vi "BuscaTeensy.vi"() -> (4 "VISA resource name out":refnum<visa-resource-name>)   [LabVIEW 2023]
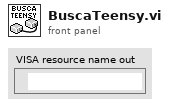
[diagram p1: front panel]
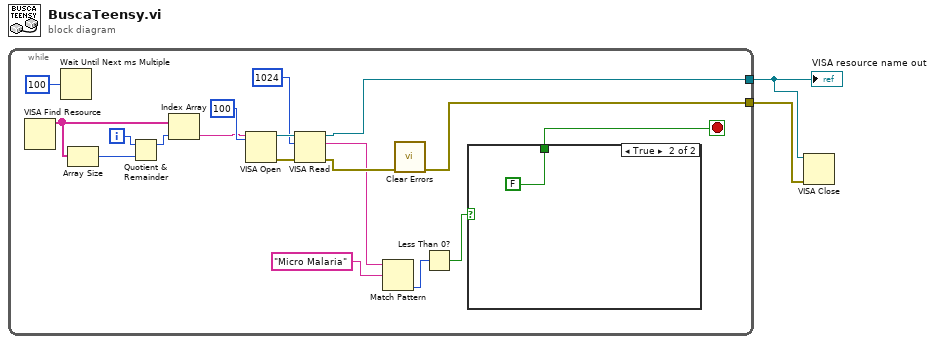
[diagram p0: block diagram]
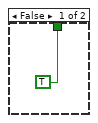
[diagram p2: hidden frame]
diagram:
  n1 = while {
    tunnel: [w11] -> w1
    tunnel: [w8] -> w2
    i -> [w15]
    stop <- w9 stop-if-true
    n2 = VISA Find Resource() -> (3:w14:string[])  [unwired: 3 in, 2 out]
    n3 = Wait Until Next ms Multiple(millisecond multiple=u32 100) -> ()  [unwired: 1 out]
    n4 = Array Size(array=w14) -> (size(s)=w16:i32)
    n5 = Quotient & Remainder(x=w15, y=w16) -> (x-y*floor(x/y)=w13:i32)  [unwired: 1 out]
    n6 = Index Array(array=w14, index=w13) -> (element=w3:string)
    n7 = VISA Open(timeout (0)=u32 100 ("VISA Open timeout (0)"), VISA resource name=w3) -> (VISA resource name=w17:refnum<visa-resource-name>, error out=w18:errorcluster)  [unwired: 3 in]
    n8 = VISA Read(VISA resource name=w17, byte count=u32 1024, error in (no error)=w18) -> (VISA resource name out=w11:refnum<visa-resource-name>, read buffer=w6:string, error out=w10:errorcluster)  [unwired: 1 out]
    n9 = Match Pattern(string=w6, regular expression="Micro Malaria" ("search string")) -> (offset past match=w4:i32)  [unwired: 1 in, 3 out]
    n10 = call <vilib>:"Clear Errors.vi"("error in (no error)"=w10) -> ("error out"=w8:errorcluster)  [unwired: 5 in, 1 out]
    n11 = Less Than 0?(x=w4) -> (x < 0?=w7:bool)
    n12 = case shown="True" w7 {
      tunnel: [TRUE FALSE] -> w9
      frame False {
      }
      frame True {
      }
    }
  }
  "VISA resource name out" <- w1
  n13 = VISA Close(VISA resource name=w1, error in (no error)=w2) -> ()  [unwired: 1 out]
